vi "ToggleAllSystems.vi"(0 "reference in":refnum<class "Facade.lvclass">, 5 "Error In":errorcluster) -> (14 "reference out":refnum<class "Facade.lvclass">, 19 "Error Out":errorcluster)   [LabVIEW 2024, in "Facade.lvclass"]
uses:
  Facade.lvclass
  Facade.lvclass/Facade.ctl
  House/House_class/House.lvclass
  Systems/SecuritySystem_class/SecuritySystem.lvclass
  Systems/MusicSystem_class/MusicSystem.lvclass
  Systems/HeatingSystem_class/HeatingSystem.lvclass
  Systems/LightingSystem_class/LightingSystem.lvclass
panel:
  # "Connector Pane"
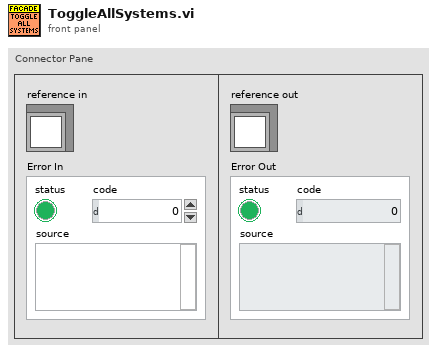
[diagram p1: front panel]
types:
  T1 = typedef "Facade.lvclass/ObjectAttributes.ctl" = cluster{"Home":refnum<class "House.lvclass">}
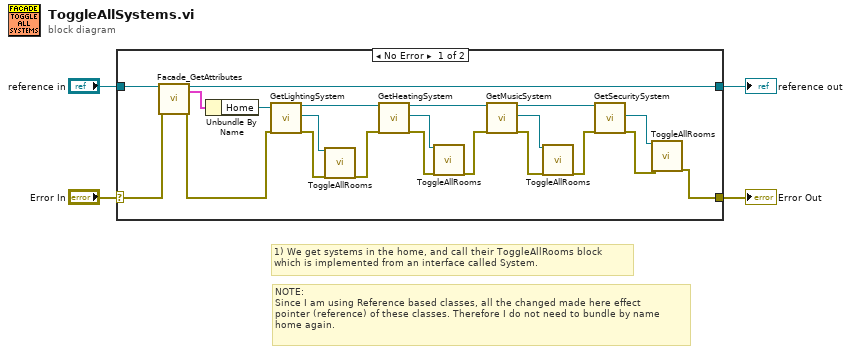
[diagram p0: block diagram]
diagram:
  # "NOTE:\nSince I am using Reference based classes, all the changed made here effect\npointer (reference) of these classes. Therefore I do not need to bundle by name\nhome again."
  # "1) We get systems in the home, and call their ToggleAllRooms block\nwhich is implemented from an interface called System."
  n1 = case shown="No Error" "Error In" {
    selector: "Error In" -> [w24 w27]
    tunnel: [w5 w27] -> w3
    tunnel: [w23 w26] -> w1
    tunnel: "reference in" -> [w25 w26]
    frame No Error {
      n2 = call "Facade_GetAttributes.vi"("reference in"=w25, "Error In"=w24) -> ("reference out"=w23:refnum<class "Facade.lvclass">, "Data"=w7:T1, "Error Out"=w6:errorcluster)  [unwired: 14 in, 1 out]
      n3 = Unbundle By Name(w7) -> ("Home"=w8:refnum<class "House.lvclass">)
      n4 = call-dynamic "GetLightingSystem.vi"("reference in"=w8, "Error In"=w6) -> ("reference out"=w22:refnum<class "House.lvclass">, "Lighting System"=w18:refnum<class "LightingSystem.lvclass">, "Error Out"=w19:errorcluster)  [unwired: 15 in]
      n5 = call-dynamic "ToggleAllRooms.vi"("reference in"=w18, "Error In"=w19) -> ("Error Out"=w17:errorcluster)  [unwired: 16 in, 1 out]
      n6 = call-dynamic "GetHeatingSystem.vi"("reference in"=w22, "Error In"=w17) -> ("reference out"=w21:refnum<class "House.lvclass">, "Heating System"=w15:refnum<class "HeatingSystem.lvclass">, "Error Out"=w16:errorcluster)  [unwired: 15 in]
      n7 = call-dynamic "ToggleAllRooms.vi"("reference in"=w15, "Error In"=w16) -> ("Error Out"=w14:errorcluster)  [unwired: 16 in, 1 out]
      n8 = call-dynamic "GetMusicSystem.vi"("reference in"=w21, "Error In"=w14) -> ("reference out"=w20:refnum<class "House.lvclass">, "Music System"=w12:refnum<class "MusicSystem.lvclass">, "Error Out"=w13:errorcluster)  [unwired: 15 in]
      n9 = call-dynamic "ToggleAllRooms.vi"("reference in"=w12, "Error In"=w13) -> ("Error Out"=w11:errorcluster)  [unwired: 16 in, 1 out]
      n10 = call-dynamic "GetSecuritySystem.vi"("reference in"=w20, "Error In"=w11) -> ("Security System"=w9:refnum<class "SecuritySystem.lvclass">, "Error Out"=w10:errorcluster)  [unwired: 15 in, 1 out]
      n11 = call-dynamic "ToggleAllRooms.vi"("reference in"=w9, "Error In"=w10) -> ("Error Out"=w5:errorcluster)  [unwired: 16 in, 1 out]
    }
    frame Error {
    }
  }
  "Error Out" <- w3
  "reference out" <- w1
